vi "WPI_IMU_ADIS16460_ReadSensorData.vi"(8 "error in (no error)":errorcluster, 11 "SPIDevRef in":T1) -> (0 "error out":errorcluster, 2 "Data Array":dbl[](array[numeric]), 3 "SPIDevRef out":T1)   [LabVIEW 2015, in "FRC ADIS16460.lvlib"]
uses:
  FRC ADIS16460.lvlib
  <vilib>/Rock Robotics/WPI/SPI/WPI_SPIDevRef.ctl
  <vilib>/Rock Robotics/SystemInterfaces/spilib/spi_bus.ctl
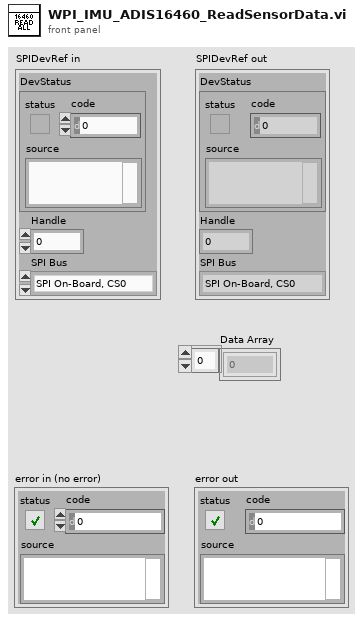
[diagram p1: front panel]
types:
  T1 = typedef "WPI_SPIDevRef.ctl" = cluster{"DevStatus":errorcluster, "Handle":i32, "SPI Bus":T2}
  T2 = typedef "spi_bus.ctl" = enum16{"SPI On-Board, CS0", "SPI On-Board, CS1", "SPI On-Board, CS2", "SPI On-Board, CS3", "SPI MXP", "Invalid"}
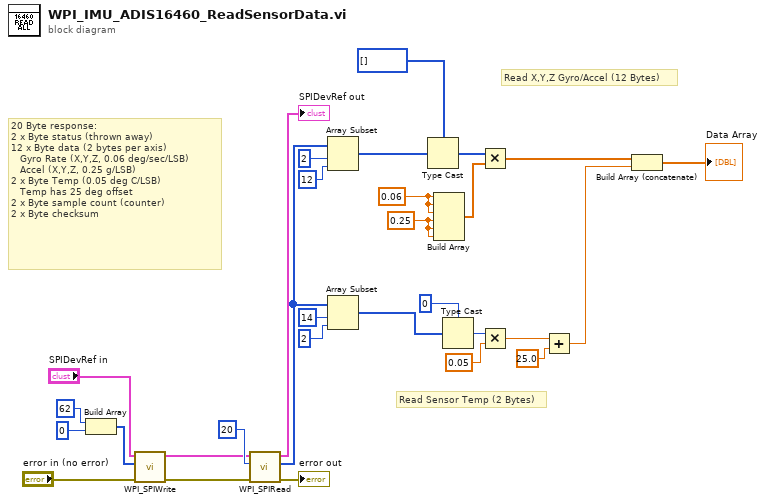
[diagram p0: block diagram]
diagram:
  w27 = 0.25
  w28 = 0.06 ("element")
  # "Read Sensor Temp (2 Bytes)"
  # "Read X,Y,Z Gyro/Accel (12 Bytes)"
  # "20 Byte response:\n2 x Byte status (thrown away)\n12 x Byte data (2 bytes per axis) \n   Gyro Rate (X,Y,Z, 0.06 deg/sec/LSB)\n   Accel (X,Y,Z, 0.25 g/LSB)\n2 x Byte Temp (0.05 deg C/LSB)\n   Temp has 25 deg offset\n2 x Byte sample count (counter)\n2 x Byte checksum"
  n1 = Build Array(u8 62 ("hi"), u8 0 ("lo")) -> (w23:u8[])
  n2 = call <vilib>:"WPI_SPIWrite.vi"("error in (no error)"="error in (no error)", "Data To Send"=w23, "SPIDevRef"="SPIDevRef in") -> ("error out"=w1:errorcluster, "SPIDevRef"=w2:T1)  [unwired: 7 out]
  n3 = call <vilib>:"WPI_SPIRead.vi"("error in (no error)"=w1, "Num to Read"=20, "SPIDevRef"=w2) -> ("error out"=→"error out":errorcluster, "Received Data"=w9:u8[], "SPIDevRef"=→"SPIDevRef out":T1)  [unwired: 6 in]
  n4 = Array Subset(array=w9, index=2, length=12) -> (w6:u8[])
  n5 = Array Subset(array=w9, index=14, length=2) -> (w10:u8[])
  n6 = Type Cast(type=i16[] [], x=w6) -> (*(type *) &x=w4:i16[])
  n7 = Build Array(w28, w28, w28, w27, w27, w27) -> (w26:dbl[])
  n8 = Type Cast(type=i16 0, x=w10) -> (*(type *) &x=w7:i16)
  n9 = Multiply(x=w4, y=w26) -> (x*y=w16:dbl[])
  n10 = Multiply(x=w7, y=0.05 ("element")) -> (x*y=w18:dbl)
  n11 = Add(x=w18, y=25.0) -> (x+y=w3:dbl)
  n12 = Build Array (concatenate)(w16, w3) -> (→"Data Array":dbl[])
